vi "MTM2_getSample_stepVectorUpdate.vi"(8 "error in (no error)":errorcluster, 11 "stepVectorUpdate_Ctl":T1={"steps[72]"=[0, 0, 0, 0, 0, 0, 0, 0, 0, 0, 0, 0, 0, 0, 0, 0, 0, 0, 0, 0, 0, 0, 0, 0, 0, 0, 0, 0, 0, 0, 0, 0, 0, 0, 0, 0, 0, 0, 0, 0, 0, 0, 0, 0, 0, 0, 0, 0, 0, 0, 0, 0, 0, 0, 0, 0, 0, 0, 0, 0, 0, 0, 0, 0, 0, 0, 0, 0, 0, 0, 0, 0]}) -> (0 "error out":errorcluster, 2 "function return":i32, 3 "stepVectorUpdate_Ctl out":T1)   [LabVIEW 2018, in "SALLV_MTM2.lvlib"]
doc: "int MTM2_shm_getSample_stepVectorUpdateLV(MTM2_stepVectorUpdateLV *stepVectorUpdate_Ctl );"
uses:
  SALLV_MTM2.lvlib
  DataTypes/stepVectorUpdate.ctl
  SALLV_MTM2.so
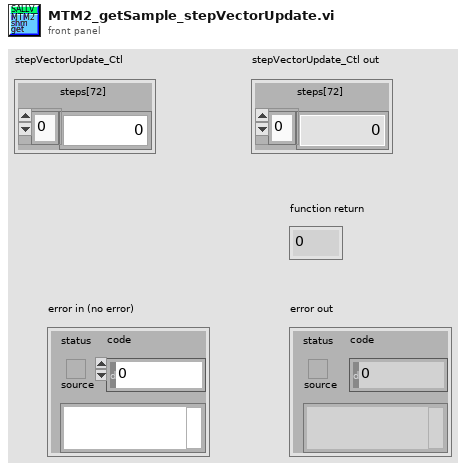
[diagram p1: front panel]
types:
  T1 = typedef "SALLV_MTM2.lvlib/stepVectorUpdate.ctl" = cluster{"steps[72]":i32[]}
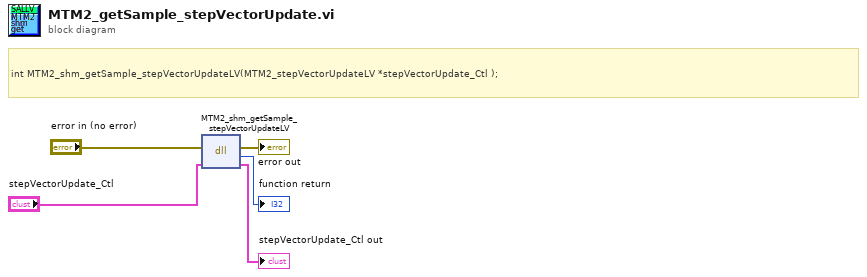
[diagram p0: block diagram]
diagram:
  # "int MTM2_shm_getSample_stepVectorUpdateLV(MTM2_stepVectorUpdateLV *stepVectorUpdate_Ctl );"
  n1 = dll-call lib="home/ttsai/Document/salApiMTM2/SALLV_MTM2/SALLV_MTM2.*" fn="MTM2_shm_getSample_stepVectorUpdateLV"(error in="error in (no error)", "stepVectorUpdate_Ctl"="stepVectorUpdate_Ctl") -> (error out=→"error out":errorcluster, →"function return":i32, "stepVectorUpdate_Ctl"=→"stepVectorUpdate_Ctl out":T1)  [unwired: 2 in, 1 out]
